vi "Pause_Initial.vi"(8 "error in (no error)":errorcluster, 10 "Blinking":bool, 11 "Reference":T1) -> (0 "error out":errorcluster, 3 "dup Reference":T1)   [LabVIEW 2025]
uses:
  Button_Reference.ctl
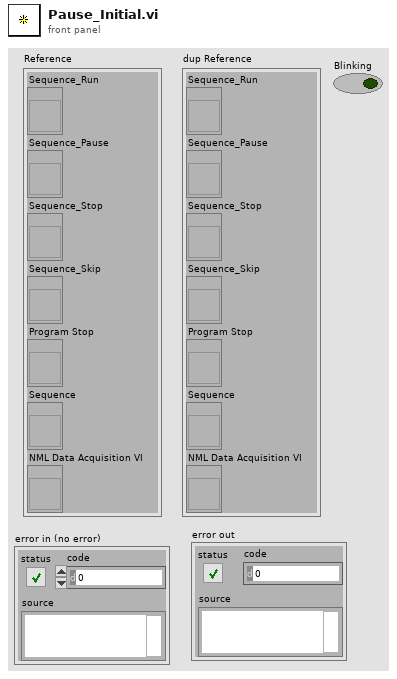
[diagram p1: front panel]
types:
  T1 = typedef "Button_Reference.ctl" = cluster{"Sequence_Run":refnum<vi>, "Sequence_Pause":refnum<vi>, "Sequence_Stop":refnum<vi>, "Sequence_Skip":refnum<vi>, "Program Stop":refnum<vi>, "Sequence":refnum<vi>, "NML Data Acquisition VI":refnum<vi>}
  T2 = enum8{"Enabled", "Disabled", "Disabled and Grayed Out"}
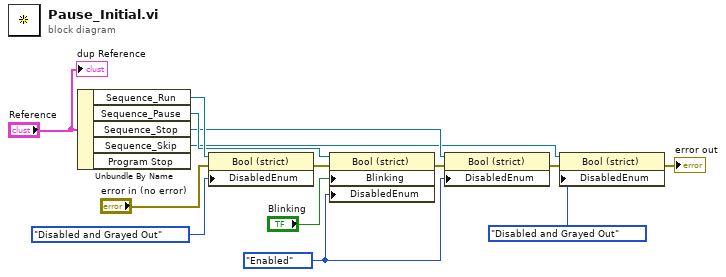
[diagram p0: block diagram]
diagram:
  w8 = T2."Enabled" ("Disabled")
  n1 = Unbundle By Name("Reference") -> ("Sequence_Run"=w5:refnum<vi>, "Sequence_Pause"=w4:refnum<vi>, "Sequence_Stop"=w3:refnum<vi>, "Sequence_Skip"=w2:refnum<vi>)  [unwired: 1 out]
  n2 = property on="Property Node" class="Bool (strict)"(reference=w5, error in="error in (no error)", "DisabledEnum"=T2."Disabled and Grayed Out" ("Disabled")) -> (error out=w12:errorcluster)  [unwired: 1 out]
  n3 = property on="Property Node" class="Bool (strict)"(reference=w4, error in=w12, "Blinking"="Blinking", "DisabledEnum"=w8) -> (error out=w13:errorcluster)  [unwired: 1 out]
  n4 = property on="Property Node" class="Bool (strict)"(reference=w3, error in=w13, "DisabledEnum"=w8) -> (error out=w14:errorcluster)  [unwired: 1 out]
  n5 = property on="Property Node" class="Bool (strict)"(reference=w2, error in=w14, "DisabledEnum"=T2."Disabled and Grayed Out" ("Disabled")) -> (error out=→"error out":errorcluster)  [unwired: 1 out]
  "dup Reference" <- "Reference"
